vi "Configure_YAxisUnit.vi"(8 "error in (no error)":errorcluster, 11 "VISA resource name":refnum<visa-resource-name>) -> (0 "error out":errorcluster)   [LabVIEW 2023, in "KeysightN9020B.lvlib"]
uses:
  KeysightN9020B.lvlib
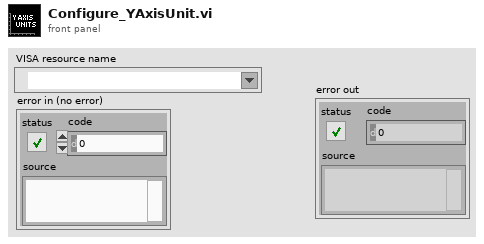
[diagram p1: front panel]
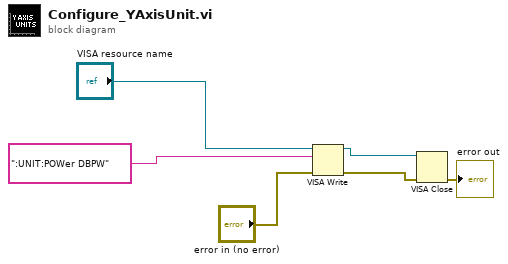
[diagram p0: block diagram]
diagram:
  n1 = VISA Write(VISA resource name="VISA resource name", write buffer=":UNIT:POWer DBPW" ("string"), error in (no error)="error in (no error)") -> (VISA resource name out=w4:refnum<visa-resource-name>, error out=w6:errorcluster)  [unwired: 1 out]
  n2 = VISA Close(VISA resource name=w4, error in (no error)=w6) -> (error out=→"error out":errorcluster)
